vi "resetFGV.vi"(8 "Write?":bool, 11 "Reset in":bool=TRUE) -> (3 "Reset out":bool)   [LabVIEW 2019]
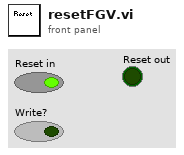
[diagram p1: front panel]
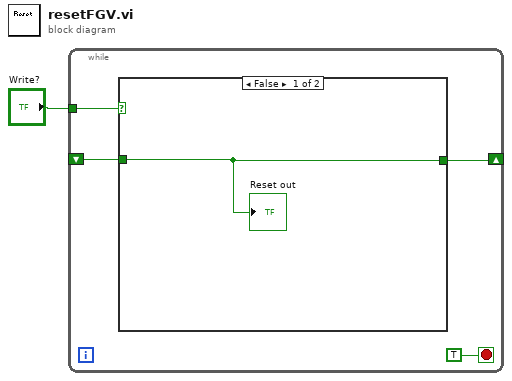
[diagram p0: block diagram]
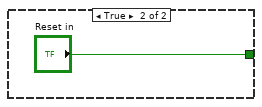
[diagram p2: hidden frame]
diagram:
  n1 = while {
    tunnel: "Write?" -> [w5]
    shift-right: [w3] -> _
    shift-left: _ -> [w2]
    stop <- TRUE stop-if-true
    n2 = case shown="False" w5 {
      tunnel: [w6 "Reset in"] -> w3
      tunnel: w2 -> [w6 _]
      frame False {
        "Reset out" <- w6
      }
      frame True {
      }
    }
  }
